vi "LED颜色分析.vi"(7 "颜色选择":enum16{"红", "绿", "蓝", "白", "黄", "琥珀色"}(ring), 8 "error in (no error)":errorcluster caption="错误输入（无错误）", 9 "分析仪通道":T1(ring), 10 "地址":string="02", 11 "MyIndex":u8) -> (0 "error out":errorcluster caption="错误输出", 2 "通道数据":u16[](array[numeric]), 3 "RGBI":string)   [LabVIEW 2015]
uses:
  <vilib>/Instr/_visa.llb/VISA Configure Serial Port (Instr).vi
panel:
  out "Read":string
  out "Send":string
  # "R"
  # "G"
  # "B"
  # "i"
  # "H"
  # "S"
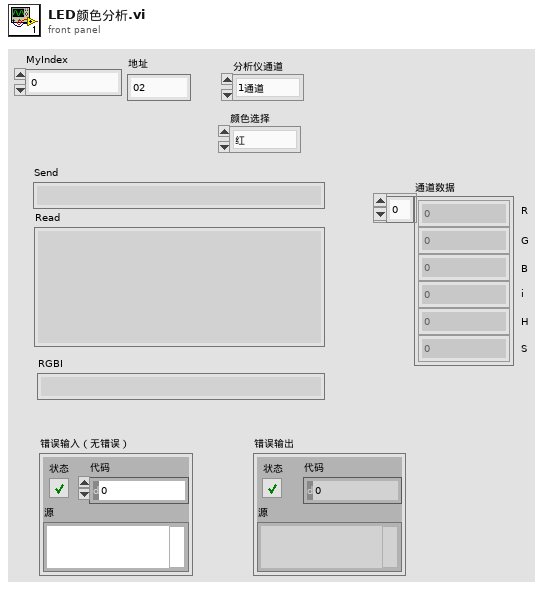
[diagram p1: front panel]
types:
  T1 = enum16{"1通道", "2通道", "3通道", "4通道", "5通道", "6通道", "7通道", "8通道", "9通道", "10通道", "11通道", "12通道", "13通道", "14通道", "15通道", "16通道"}
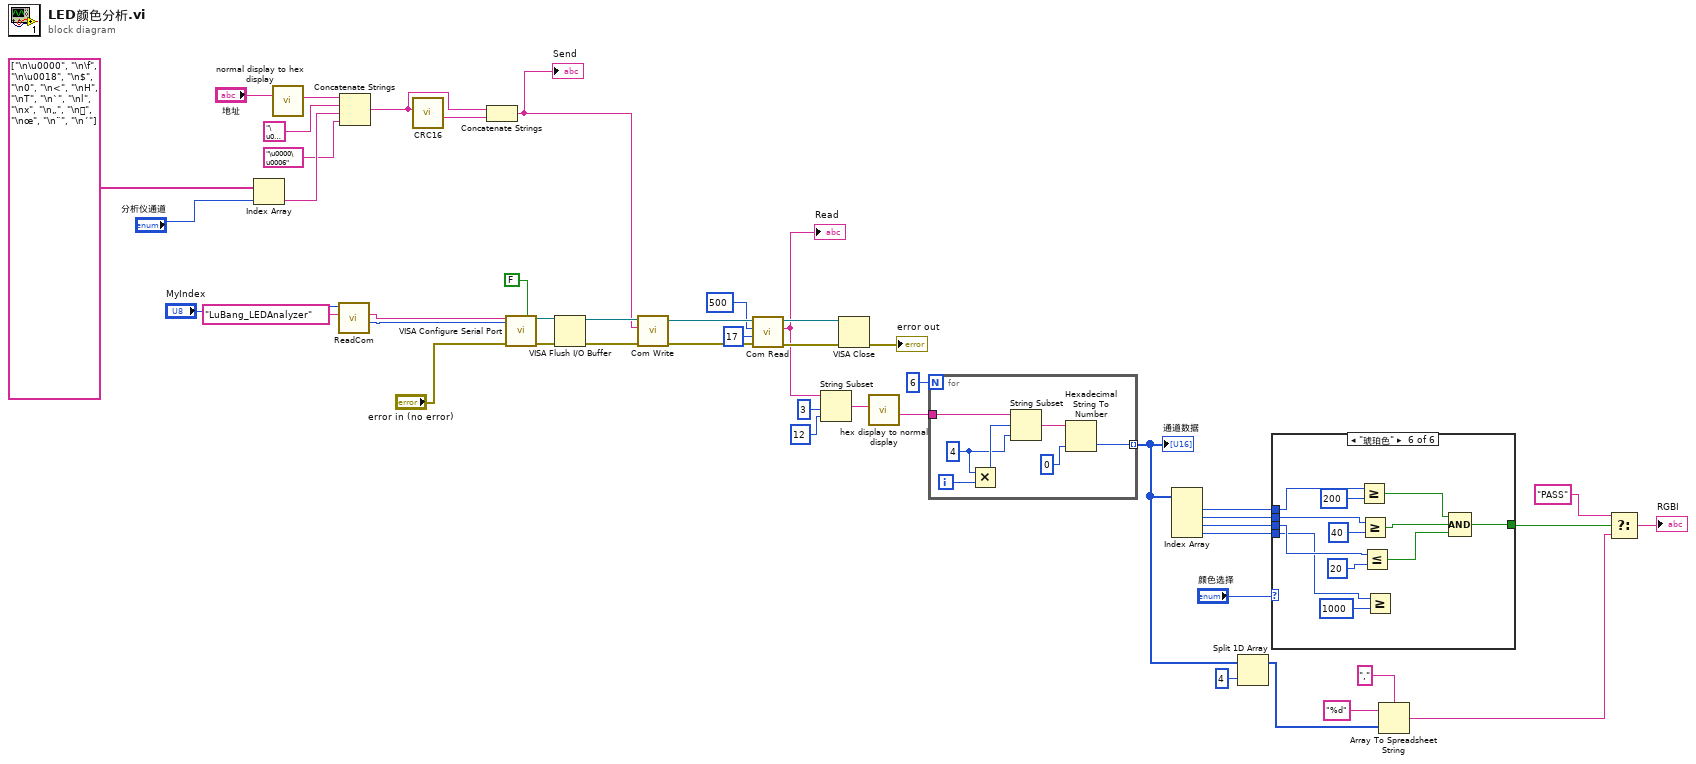
[diagram p0: block diagram]
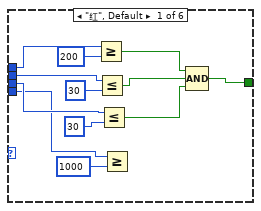
[diagram p2: hidden frame]
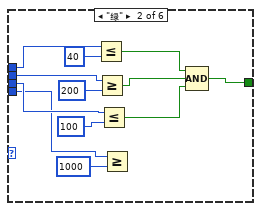
[diagram p3: hidden frame]
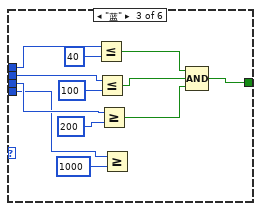
[diagram p4: hidden frame]
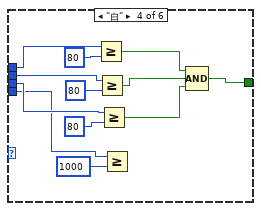
[diagram p5: hidden frame]
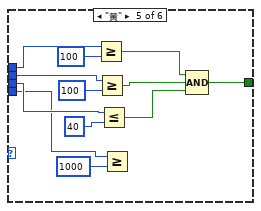
[diagram p6: hidden frame]
diagram:
  n1 = Index Array(array=string[] ["\n\u0000", "\n\f", "\n\u0018", "\n$", "\n0", "\n<", "\nH", "\nT", "\n`", "\nl", "\nx", "\n„", "\n", "\nœ", "\n¨", "\n´"], index="分析仪通道") -> (element=w36:string)
  n2 = call "normal display to hex display.vi"("Normal display"="地址") -> ("Hex display"=w40:string)  [unwired: 6 in]
  n3 = call "ReadCom.vi"("仪器名称"="LuBang_LEDAnalyzer", "MyIndex"="MyIndex") -> ("Baudrate"=w1:i32, "COM"=w2:string)  [unwired: 7 in, 1 out]
  n4 = Concatenate Strings(w40, "\u0003", w36, "\u0000\u0006") -> (w44:string)
  n5 = call "CRC16.vi"("输入字符串"=w44) -> ("CRC16(String)"=w43:string)  [unwired: 9 in, 1 out]
  n6 = Concatenate Strings(w44, w43) -> (w32:string)
  "Send" <- w32
  n7 = call-poly "VISA Configure Serial Port"("VISA resource name"=w2, "Enable Termination\nChar (T)"=FALSE ("Enable Termination\nChar (T)"), "baud rate (9600)"=w1, "error in (no error)"="error in (no error)") -> ("VISA resource name out"=w45:refnum<visa-resource-name>, "error out"=w46:errorcluster)  [unwired: 10 in]
  n8 = VISA Flush I/O Buffer(VISA resource name=w45, error in (no error)=w46) -> (VISA resource name out=w34:refnum<visa-resource-name>, error out=w33:errorcluster)  [unwired: 1 in]
  n9 = call "Com Write.vi"("错误输入（无错误）"=w33, "Wbuff"=w32, "VISA In"=w34) -> ("错误输出"=w31:errorcluster, "VISA Out"=w30:refnum<visa-resource-name>)  [unwired: 7 in]
  n10 = call "Com Read.vi"("错误输入（无错误）"=w31, "num"=u32 17, "超时"=u32 500, "VISA In"=w30) -> ("错误输出"=w26:errorcluster, "buff"=w25:string, "VISA Out"=w27:refnum<visa-resource-name>)  [unwired: 5 in]
  "Read" <- w25
  n11 = String Subset(string=w25, offset (0)=3 ("长度（剩余）"), length (rest)=12 ("长度（剩余）")) -> (substring=w22:string)
  n12 = VISA Close(VISA resource name=w27, error in (no error)=w26) -> (error out=→"error out":errorcluster)
  n13 = call "hex display to normal display.vi"("Hex display"=w22) -> ("Normal display"=w21:string)  [unwired: 10 in]
  n14 = for {
    N: 6 -> [_]
    tunnel: w21 -> [w54]
    tunnel: [w49] -> w6 mode=indexing
    i -> [w53]
    w51 = 4
    n15 = Multiply(x=w51, y=w53) -> (x*y=w52:i32)
    n16 = String Subset(string=w54, offset (0)=w52, length (rest)=w51) -> (substring=w50:string)
    n17 = Hexadecimal String To Number(string=w50, default (0uL)=u16 0) -> (number=w49:u16)  [unwired: 1 in, 1 out]
  }
  "通道数据" <- w6
  n18 = Index Array(array=w6) -> (element #1=w18:u16, element #2=w17:u16, element #3=w16:u16, element #4=w15:u16)  [unwired: 4 in]
  n19 = Split 1D Array(array=w6, index=4 ("索引")) -> (first subarray=w8:u16[])  [unwired: 1 out]
  n20 = case shown="\"琥珀色\"" "颜色选择" {
    tunnel: w18 -> [w66 w78 w90 w102 w114 w126]
    tunnel: w17 -> [w64 w76 w88 w100 w112 w124]
    tunnel: w16 -> [w62 w74 w86 w98 w110 w122]
    tunnel: w15 -> [w56 w68 w80 w92 w104 w116]
    tunnel: [w57 w69 w81 w93 w105 w117] -> w14
    frame "红", Default {
      n21 = Greater Or Equal?(x=w66, y=u32 200) -> (x >= y?=w60:bool)
      n22 = Less Or Equal?(x=w64, y=u32 30) -> (x <= y?=w59:bool)
      n23 = Less Or Equal?(x=w62, y=u32 30) -> (x <= y?=w58:bool)
      n24 = Greater Or Equal?(x=w56, y=u32 1000) -> ()  [unwired: 1 out]
      n25 = Compound Arithmetic op=AND ("复合运算")(w60, w59, w58) -> (w57:bool)
    }
    frame "绿" {
      n26 = Less Or Equal?(x=w78, y=u32 40) -> (x <= y?=w72:bool)
      n27 = Greater Or Equal?(x=w76, y=u32 200) -> (x >= y?=w71:bool)
      n28 = Less Or Equal?(x=w74, y=u32 100) -> (x <= y?=w70:bool)
      n29 = Greater Or Equal?(x=w68, y=u32 1000) -> ()  [unwired: 1 out]
      n30 = Compound Arithmetic op=AND ("复合运算")(w72, w71, w70) -> (w69:bool)
    }
    frame "蓝" {
      n31 = Less Or Equal?(x=w90, y=u32 40) -> (x <= y?=w84:bool)
      n32 = Less Or Equal?(x=w88, y=u32 100) -> (x <= y?=w83:bool)
      n33 = Greater Or Equal?(x=w86, y=u32 200) -> (x >= y?=w82:bool)
      n34 = Greater Or Equal?(x=w80, y=u32 1000) -> ()  [unwired: 1 out]
      n35 = Compound Arithmetic op=AND ("复合运算")(w84, w83, w82) -> (w81:bool)
    }
    frame "白" {
      n36 = Greater Or Equal?(x=w102, y=u32 80) -> (x >= y?=w96:bool)
      n37 = Greater Or Equal?(x=w100, y=u32 80) -> (x >= y?=w95:bool)
      n38 = Greater Or Equal?(x=w98, y=u32 80) -> (x >= y?=w94:bool)
      n39 = Greater Or Equal?(x=w92, y=u32 1000) -> ()  [unwired: 1 out]
      n40 = Compound Arithmetic op=AND ("复合运算")(w96, w95, w94) -> (w93:bool)
    }
    frame "黄" {
      n41 = Greater Or Equal?(x=w114, y=u32 100) -> (x >= y?=w108:bool)
      n42 = Greater Or Equal?(x=w112, y=u32 100) -> (x >= y?=w107:bool)
      n43 = Less Or Equal?(x=w110, y=u32 40) -> (x <= y?=w106:bool)
      n44 = Greater Or Equal?(x=w104, y=u32 1000) -> ()  [unwired: 1 out]
      n45 = Compound Arithmetic op=AND ("复合运算")(w108, w107, w106) -> (w105:bool)
    }
    frame "琥珀色" {
      n46 = Greater Or Equal?(x=w126, y=u32 200) -> (x >= y?=w120:bool)
      n47 = Greater Or Equal?(x=w124, y=u32 40) -> (x >= y?=w119:bool)
      n48 = Less Or Equal?(x=w122, y=u32 20) -> (x <= y?=w118:bool)
      n49 = Greater Or Equal?(x=w116, y=u32 1000) -> ()  [unwired: 1 out]
      n50 = Compound Arithmetic op=AND ("复合运算")(w120, w119, w118) -> (w117:bool)
    }
  }
  n51 = Array To Spreadsheet String(delimiter (Tab)="," ("分隔符(Tab)"), array=w8, 3:"%d") -> (spreadsheet string=w7:string)
  n52 = Select(t="PASS", s=w14, f=w7) -> (s? t:f=→"RGBI":string)
